vi "Logger Control.vi"(10 "Command":T1=enum."Start") -> (2 "notifier out":refnum<notifier>)   [LabVIEW 2015]
uses:
  Logger Command.ctl
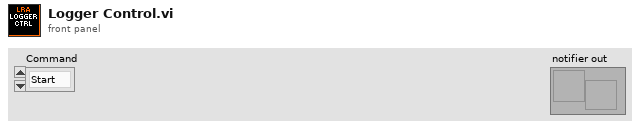
[diagram p1: front panel]
types:
  T1 = typedef "Logger Command.ctl" = enum16{"Init", "Start", "Stop"}
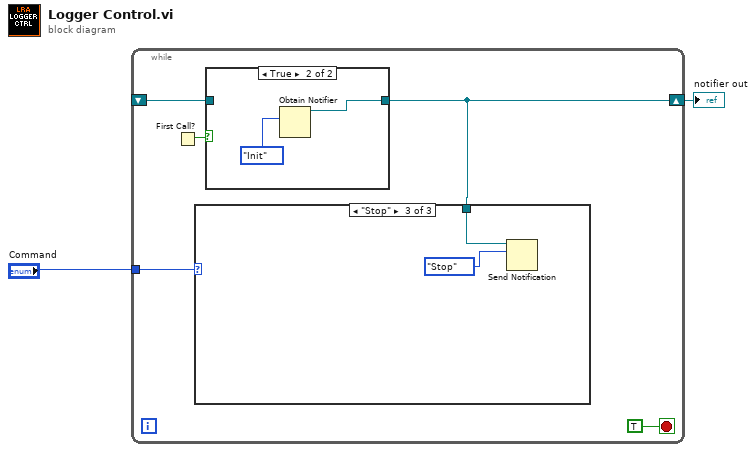
[diagram p0: block diagram]
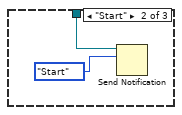
[diagram p3: hidden frame]
diagram:
  n1 = while {
    shift-right: [w3] -> w1
    shift-left: _ -> [w5]
    tunnel: "Command" -> [w4]
    stop <- TRUE stop-if-true
    n2 = First Call?() -> (First Call?: T/F=w6:bool)
    n3 = case shown="True" w6 {
      tunnel: [w12 w14] -> w3
      tunnel: w5 -> [w12 _]
      frame False {
      }
      frame True {
        n4 = Obtain Notifier(notification data type=Logger_Command."Init" ("Command")) -> (notifier out=w14:refnum<notifier>)  [unwired: 3 in, 2 out]
      }
    }
    n5 = case shown="\"Stop\"" w4 {
      tunnel: w3 -> [_ w9 w11]
      frame "Init", Default {
      }
      frame "Start" {
        n6 = Send Notification(notification=Logger_Command."Start", notifier=w9) -> ()  [unwired: 1 in, 2 out]
      }
      frame "Stop" {
        n7 = Send Notification(notification=Logger_Command."Stop", notifier=w11) -> ()  [unwired: 1 in, 2 out]
      }
    }
  }
  "notifier out" <- w1
